vi "PathPlanner_IdealStartingState_New.vi"(9 "Rotation":T1={"VALUE"=0.0, "COS"=1.0, "SIN"=0.0} {"SIN" format="%13.4f"; "COS" format="%13.4f"; "VALUE" format="%13.4f"}, 11 "VelocityMPS":dbl) -> (3 "IdealStartingState":T2={"VelocityMPS"=0.0, "Rotation"={"VALUE"=0.0, "COS"=1.0, "SIN"=0.0}, "NotNull"=FALSE} {"Rotation"."SIN" format="%13.4f"; "Rotation"."COS" format="%13.4f"; "Rotation"."VALUE" format="%13.4f"})   [LabVIEW 2019, in "PathPlanner24.lvlib"]
doc: "Describes the ideal starting state of the robot when starting a path\n\nInputs: \n -- velocityMPS - double - The ideal starting velocity (M/S)\n -- rotation - Rotation2d - The ideal starting rotation\n\nOutputs:\n -- IdealStartingState - cluster - data structure"
uses:
  PathPlanner24.lvlib
  TypeDef/PathPlannerIdealStartingState.ctl
  <vilib>/Rock Robotics/WPI/ThirdParty/JAS_Junk/TrajLib/TypeDef/ROTATION2D.ctl
  <vilib>/Rock Robotics/WPI/ThirdParty/JAS_Junk/TrajLib/Trajectory_Library.lvlib
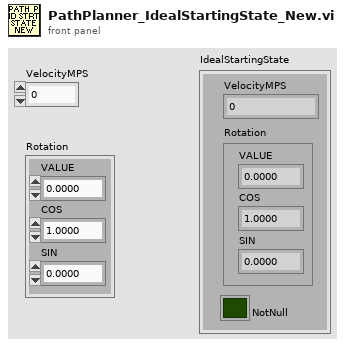
[diagram p1: front panel]
types:
  T1 = typedef "Trajectory_Library.lvlib/ROTATION2D.ctl" = cluster{"VALUE":dbl, "COS":dbl, "SIN":dbl}
  T2 = typedef "PathPlanner24.lvlib/PathPlannerIdealStartingState.ctl" = cluster{"VelocityMPS":dbl, "Rotation":T1, "NotNull":bool}
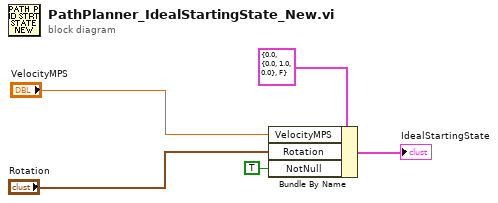
[diagram p0: block diagram]
diagram:
  n1 = Bundle By Name(cluster=T2 {"VelocityMPS"=0.0, "Rotation"={"VALUE"=0.0, "COS"=1.0, "SIN"=0.0}, "NotNull"=FALSE} ("IdealStartingState"), "VelocityMPS"="VelocityMPS", "Rotation"="Rotation", "NotNull"=TRUE) -> (→"IdealStartingState":T2)
